vi "Dut Rx Initiate.vi"(0 "MTK7615 in":refnum<class "MTK7615.lvclass">, 11 "error in (no error)":errorcluster) -> (4 "MTK7615 out":refnum<class "MTK7615.lvclass">, 15 "error out":errorcluster)   [LabVIEW 2015, in "MTK7615.lvlib" / "MTK7615.lvclass"]
uses:
  MTK7615.lvclass
  Technologies/WLAN/Dut/Objects/BASE_class/niDTS WLAN Dut.lvclass
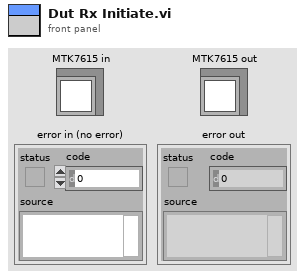
[diagram p1: front panel]
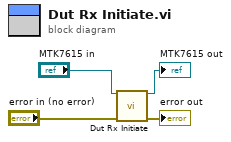
[diagram p0: block diagram]
diagram:
  n1 = call-parent "Dut Rx Initiate.vi"("niDTS DUT in"="MTK7615 in", "error in (no error)"="error in (no error)") -> ("niDTS DUT out"=→"MTK7615 out":refnum<class "MTK7615.lvclass">, "error out"=→"error out":errorcluster)  [unwired: 12 in]
